vi "MCSC_4CH_4.04.vi"() -> ()   [LabVIEW 2012]
uses:
  <vilib>/Analysis/baseanly.llb/Mean (DBL).vi
  Libraries and VIs/Scalar_Data_4.vi
  Libraries and VIs/Scalar_Data_3.vi
  Libraries and VIs/Scalar_Data_2.vi
  Libraries and VIs/Scalar_Data.vi
  AmcsUsb.dll
  <vilib>/Analysis/NI_AALBase.lvlib
panel:
  in  "y":dbl
  in  "Data Reads":i32=962
  out "Loop Count":i32=961
  in  "TC Start":i32=100 min=100 max=1894
  in  "TC Length":i32=1894 min=100 max=1894
  out "Total Counts":cluster{dbl, dbl, dbl, dbl}(graph)={27003.0, 22784.0, 0.0, 0.0}
  out "return type":i32
  out "Raw Uncorrected Return":dbl[][](graph)=[[20897.0, 50029.0, 450.0, 783.0, 1128.0, 1525.0, 1812.0, 1978.0, 1912.0, 1724.0, 1571.0, 1324.0, 1184.0, 1034.0, 915.0, 833.0, 773.0, 692.0, 623.0, 619.0, 486.0, 513.0, 479.0, 406.0, 417.0, 375.0, 341.0, 359.0, 321.0, 307.0, 290.0, 262.0, 248.0, 258.0, 190.0, 213.0, 203.0, 200.0, 203.0, 201.0, 156.0, 159.0, 181.0, 160.0, 179.0, 176.0, 175.0, 192.0, 163.0, 145.0, 185.0, 176.0, 166.0, 155.0, 167.0, 159.0, 149.0, 154.0, 232.0, 335.0, 318.0, 198.0, 164.0, 167.0, 148.0, 145.0, 151.0, 129.0, 173.0, 165.0, 139.0, 150.0, 165.0, 157.0, 165.0, 158.0, 144.0, 160.0, 163.0, 159.0, 146.0, 139.0, 136.0, 134.0, 168.0, 141.0, 123.0, 160.0, 142.0, 151.0, 159.0, 167.0, 145.0, 160.0, 154.0, 144.0, 150.0, 157.0, 146.0, 146.0, 143.0, 171.0, 165.0, 142.0, 149.0, 150.0, 158.0, 148.0, 153.0, 142.0, 142.0, 141.0, 174.0, 141.0, 161.0, 163.0, 144.0, 134.0, 136.0, 142.0, 148.0, 140.0, 157.0, 172.0, 167.0, 152.0, 147.0, 137.0, 166.0, 149.0, 135.0, 132.0, 142.0, 142.0, 140.0, 148.0, 163.0, 160.0, 130.0, 130.0, 162.0, 174.0, 153.0, 157.0, 154.0, 171.0, 152.0, 160.0, 150.0, 180.0, 139.0, 140.0, 156.0, 148.0, 141.0, 158.0, 157.0, 133.0, 166.0, 146.0, 146.0, 150.0, 138.0, 133.0, 165.0, 153.0, 133.0, 128.0, 129.0, 157.0, 154.0, 136.0, 145.0, 159.0, 142.0, 131.0, 133.0, 148.0, 165.0, 143.0, 143.0, 135.0, 134.0, 151.0, 179.0, 166.0, 144.0, 151.0, 166.0, 152.0, 156.0, 150.0, 160.0, 130.0, 164.0, 147.0, 155.0, 129.0, 164.0, 163.0, 163.0, 133.0, 182.0, 153.0, 128.0, 151.0, 157.0, 144.0, 180.0, 129.0, 148.0, 136.0, 144.0, 150.0, 146.0, 145.0, 163.0, 146.0, 158.0, 150.0, 154.0, 180.0, 152.0, 152.0, 153.0, 148.0, 158.0, 152.0, 161.0, 154.0, 151.0, 124.0, 133.0, 143.0, 154.0, 134.0, 144.0, 152.0, 150.0, 161.0, 148.0, 156.0, 129.0, 162.0, 157.0, 154.0, 167.0, 149.0, 159.0, 170.0, 155.0, 158.0, 137.0, 149.0, 155.0, 149.0, 129.0, 156.0, 140.0, 170.0, 172.0, 149.0, 142.0, 153.0, 146.0, 152.0, 155.0, 143.0, 115.0, 135.0, 155.0, 145.0, 136.0, 154.0, 146.0, 161.0, 144.0, 170.0, 148.0, 137.0], [142.0, 41325.0, 486.0, 804.0, 1162.0, 1626.0, 1885.0, 1884.0, 1837.0, 1564.0, 1349.0, 1108.0, 1006.0, 860.0, 746.0, 643.0, 549.0, 466.0, 456.0, 433.0, 335.0, 343.0, 328.0, 255.0, 264.0, 235.0, 239.0, 222.0, 207.0, 180.0, 170.0, 159.0, 175.0, 169.0, 158.0, 168.0, 161.0, 154.0, 160.0, 166.0, 139.0, 124.0, 134.0, 165.0, 114.0, 120.0, 158.0, 144.0, 141.0, 127.0, 121.0, 126.0, 130.0, 128.0, 136.0, 115.0, 148.0, 132.0, 153.0, 178.0, 163.0, 145.0, 129.0, 124.0, 111.0, 115.0, 142.0, 128.0, 127.0, 157.0, 139.0, 135.0, 137.0, 148.0, 112.0, 119.0, 122.0, 137.0, 110.0, 140.0, 132.0, 135.0, 158.0, 151.0, 122.0, 123.0, 122.0, 130.0, 127.0, 134.0, 139.0, 140.0, 124.0, 116.0, 134.0, 129.0, 120.0, 138.0, 124.0, 129.0, 152.0, 115.0, 121.0, 113.0, 108.0, 126.0, 119.0, 133.0, 132.0, 134.0, 147.0, 126.0, 134.0, 101.0, 122.0, 130.0, 130.0, 128.0, 128.0, 131.0, 122.0, 118.0, 113.0, 135.0, 118.0, 128.0, 114.0, 128.0, 137.0, 148.0, 114.0, 116.0, 139.0, 129.0, 116.0, 123.0, 132.0, 128.0, 119.0, 123.0, 120.0, 115.0, 135.0, 127.0, 98.0, 115.0, 118.0, 110.0, 120.0, 100.0, 132.0, 131.0, 134.0, 126.0, 131.0, 131.0, 135.0, 116.0, 137.0, 131.0, 135.0, 118.0, 121.0, 109.0, 129.0, 126.0, 110.0, 85.0, 116.0, 126.0, 134.0, 122.0, 143.0, 132.0, 116.0, 136.0, 120.0, 128.0, 120.0, 130.0, 123.0, 139.0, 120.0, 112.0, 125.0, 123.0, 145.0, 127.0, 121.0, 141.0, 122.0, 128.0, 122.0, 127.0, 123.0, 119.0, 126.0, 133.0, 113.0, 124.0, 147.0, 126.0, 139.0, 124.0, 122.0, 108.0, 136.0, 129.0, 137.0, 151.0, 127.0, 129.0, 138.0, 104.0, 123.0, 132.0, 120.0, 132.0, 127.0, 132.0, 128.0, 123.0, 134.0, 137.0, 121.0, 135.0, 131.0, 123.0, 153.0, 134.0, 119.0, 120.0, 123.0, 124.0, 117.0, 116.0, 132.0, 120.0, 124.0, 135.0, 135.0, 131.0, 128.0, 132.0, 113.0, 133.0, 127.0, 136.0, 137.0, 116.0, 133.0, 132.0, 130.0, 131.0, 141.0, 127.0, 145.0, 127.0, 129.0, 112.0, 137.0, 126.0, 128.0, 134.0, 122.0, 137.0, 120.0, 131.0, 146.0, 153.0, 134.0, 125.0, 109.0, 110.0, 130.0, 134.0, 130.0, 128.0, 136.0, 126.0], [145.0, 0.0, 0.0, 0.0, 0.0, 0.0, 0.0, 0.0, 0.0, 0.0, 0.0, 0.0, 0.0, 0.0, 0.0, 0.0, 0.0, 0.0, 0.0, 0.0, 0.0, 0.0, 0.0, 0.0, 0.0, 0.0, 0.0, 0.0, 0.0, 0.0, 0.0, 0.0, 0.0, 0.0, 0.0, 0.0, 0.0, 0.0, 0.0, 0.0, 0.0, 0.0, 0.0, 0.0, 0.0, 0.0, 0.0, 0.0, 0.0, 0.0, 0.0, 0.0, 0.0, 0.0, 0.0, 0.0, 0.0, 0.0, 0.0, 0.0, 0.0, 0.0, 0.0, 0.0, 0.0, 0.0, 0.0, 0.0, 0.0, 0.0, 0.0, 0.0, 0.0, 0.0, 0.0, 0.0, 0.0, 0.0, 0.0, 0.0, 0.0, 0.0, 0.0, 0.0, 0.0, 0.0, 0.0, 0.0, 0.0, 0.0, 0.0, 0.0, 0.0, 0.0, 0.0, 0.0, 0.0, 0.0, 0.0, 0.0, 0.0, 0.0, 0.0, 0.0, 0.0, 0.0, 0.0, 0.0, 0.0, 0.0, 0.0, 0.0, 0.0, 0.0, 0.0, 0.0, 0.0, 0.0, 0.0, 0.0, 0.0, 0.0, 0.0, 0.0, 0.0, 0.0, 0.0, 0.0, 0.0, 0.0, 0.0, 0.0, 0.0, 0.0, 0.0, 0.0, 0.0, 0.0, 0.0, 0.0, 0.0, 0.0, 0.0, 0.0, 0.0, 0.0, 0.0, 0.0, 0.0, 0.0, 0.0, 0.0, 0.0, 0.0, 0.0, 0.0, 0.0, 0.0, 0.0, 0.0, 0.0, 0.0, 0.0, 0.0, 0.0, 0.0, 0.0, 0.0, 0.0, 0.0, 0.0, 0.0, 0.0, 0.0, 0.0, 0.0, 0.0, 0.0, 0.0, 0.0, 0.0, 0.0, 0.0, 0.0, 0.0, 0.0, 0.0, 0.0, 0.0, 0.0, 0.0, 0.0, 0.0, 0.0, 0.0, 0.0, 0.0, 0.0, 0.0, 0.0, 0.0, 0.0, 0.0, 0.0, 0.0, 0.0, 0.0, 0.0, 0.0, 0.0, 0.0, 0.0, 0.0, 0.0, 0.0, 0.0, 0.0, 0.0, 0.0, 0.0, 0.0, 0.0, 0.0, 0.0, 0.0, 0.0, 0.0, 0.0, 0.0, 0.0, 0.0, 0.0, 0.0, 0.0, 0.0, 0.0, 0.0, 0.0, 0.0, 0.0, 0.0, 0.0, 0.0, 0.0, 0.0, 0.0, 0.0, 0.0, 0.0, 0.0, 0.0, 0.0, 0.0, 0.0, 0.0, 0.0, 0.0, 0.0, 0.0, 0.0, 0.0, 0.0, 0.0, 0.0, 0.0, 0.0, 0.0, 0.0, 0.0, 0.0, 0.0, 0.0, 0.0, 0.0, 0.0, 0.0, 0.0, 0.0, 0.0, 0.0], [0.0, 0.0, 0.0, 0.0, 0.0, 0.0, 0.0, 0.0, 0.0, 0.0, 0.0, 0.0, 0.0, 0.0, 0.0, 0.0, 0.0, 0.0, 0.0, 0.0, 0.0, 0.0, 0.0, 0.0, 0.0, 0.0, 0.0, 0.0, 0.0, 0.0, 0.0, 0.0, 0.0, 0.0, 0.0, 0.0, 0.0, 0.0, 0.0, 0.0, 0.0, 0.0, 0.0, 0.0, 0.0, 0.0, 0.0, 0.0, 0.0, 0.0, 0.0, 0.0, 0.0, 0.0, 0.0, 0.0, 0.0, 0.0, 0.0, 0.0, 0.0, 0.0, 0.0, 0.0, 0.0, 0.0, 0.0, 0.0, 0.0, 0.0, 0.0, 0.0, 0.0, 0.0, 0.0, 0.0, 0.0, 0.0, 0.0, 0.0, 0.0, 0.0, 0.0, 0.0, 0.0, 0.0, 0.0, 0.0, 0.0, 0.0, 0.0, 0.0, 0.0, 0.0, 0.0, 0.0, 0.0, 0.0, 0.0, 0.0, 0.0, 0.0, 0.0, 0.0, 0.0, 0.0, 0.0, 0.0, 0.0, 0.0, 0.0, 0.0, 0.0, 0.0, 0.0, 0.0, 0.0, 0.0, 0.0, 0.0, 0.0, 0.0, 0.0, 0.0, 0.0, 0.0, 0.0, 0.0, 0.0, 0.0, 0.0, 0.0, 0.0, 0.0, 0.0, 0.0, 0.0, 0.0, 0.0, 0.0, 0.0, 0.0, 0.0, 0.0, 0.0, 0.0, 0.0, 0.0, 0.0, 0.0, 0.0, 0.0, 0.0, 0.0, 0.0, 0.0, 0.0, 0.0, 0.0, 0.0, 0.0, 0.0, 0.0, 0.0, 0.0, 0.0, 0.0, 0.0, 0.0, 0.0, 0.0, 0.0, 0.0, 0.0, 0.0, 0.0, 0.0, 0.0, 0.0, 0.0, 0.0, 0.0, 0.0, 0.0, 0.0, 0.0, 0.0, 0.0, 0.0, 0.0, 0.0, 0.0, 0.0, 0.0, 0.0, 0.0, 0.0, 0.0, 0.0, 0.0, 0.0, 0.0, 0.0, 0.0, 0.0, 0.0, 0.0, 0.0, 0.0, 0.0, 0.0, 0.0, 0.0, 0.0, 0.0, 0.0, 0.0, 0.0, 0.0, 0.0, 0.0, 0.0, 0.0, 0.0, 0.0, 0.0, 0.0, 0.0, 0.0, 0.0, 0.0, 0.0, 0.0, 0.0, 0.0, 0.0, 0.0, 0.0, 0.0, 0.0, 0.0, 0.0, 0.0, 0.0, 0.0, 0.0, 0.0, 0.0, 0.0, 0.0, 0.0, 0.0, 0.0, 0.0, 0.0, 0.0, 0.0, 0.0, 0.0, 0.0, 0.0, 0.0, 0.0, 0.0, 0.0, 0.0, 0.0, 0.0, 0.0, 0.0, 0.0, 0.0, 0.0, 0.0, 0.0, 0.0, 0.0, 0.0, 0.0, 0.0]]
  in  "stop":bool
  out "Corrected Return":dbl[][](graph)=[[20749.1, 49881.1, 302.1, 635.1, 980.1, 1377.1, 1664.1, 1830.1, 1764.1, 1576.1, 1423.1, 1176.1, 1036.1, 886.1, 767.1, 685.1, 625.1, 544.1, 475.1, 471.1, 338.1, 365.1, 331.1, 258.1, 269.1, 227.1, 193.1, 211.1, 173.1, 159.1, 142.1, 114.1, 100.1, 110.1, 42.099999999999994, 65.1, 55.099999999999994, 52.099999999999994, 55.099999999999994, 53.099999999999994, 8.099999999999994, 11.099999999999994, 33.099999999999994, 12.099999999999994, 31.099999999999994, 28.099999999999994, 27.099999999999994, 44.099999999999994, 15.099999999999994, -2.9000000000000057, 37.099999999999994, 28.099999999999994, 18.099999999999994, 7.099999999999994, 19.099999999999994, 11.099999999999994, 1.0999999999999943, 6.099999999999994, 84.1, 187.1, 170.1, 50.099999999999994, 16.099999999999994, 19.099999999999994, 0.09999999999999432, -2.9000000000000057, 3.0999999999999943, -18.900000000000006, 25.099999999999994, 17.099999999999994, -8.900000000000006, 2.0999999999999943, 17.099999999999994, 9.099999999999994, 17.099999999999994, 10.099999999999994, -3.9000000000000057, 12.099999999999994, 15.099999999999994, 11.099999999999994, -1.9000000000000057, -8.900000000000006, -11.900000000000006, -13.900000000000006, 20.099999999999994, -6.900000000000006, -24.900000000000006, 12.099999999999994, -5.900000000000006, 3.0999999999999943, 11.099999999999994, 19.099999999999994, -2.9000000000000057, 12.099999999999994, 6.099999999999994, -3.9000000000000057, 2.0999999999999943, 9.099999999999994, -1.9000000000000057, -1.9000000000000057, -4.900000000000006, 23.099999999999994, 17.099999999999994, -5.900000000000006, 1.0999999999999943, 2.0999999999999943, 10.099999999999994, 0.09999999999999432, 5.099999999999994, -5.900000000000006, -5.900000000000006, -6.900000000000006, 26.099999999999994, -6.900000000000006, 13.099999999999994, 15.099999999999994, -3.9000000000000057, -13.900000000000006, -11.900000000000006, -5.900000000000006, 0.09999999999999432, -7.900000000000006, 9.099999999999994, 24.099999999999994, 19.099999999999994, 4.099999999999994, -0.9000000000000057, -10.900000000000006, 18.099999999999994, 1.0999999999999943, -12.900000000000006, -15.900000000000006, -5.900000000000006, -5.900000000000006, -7.900000000000006, 0.09999999999999432, 15.099999999999994, 12.099999999999994, -17.900000000000006, -17.900000000000006, 14.099999999999994, 26.099999999999994, 5.099999999999994, 9.099999999999994, 6.099999999999994, 23.099999999999994, 4.099999999999994, 12.099999999999994, 2.0999999999999943, 32.099999999999994, -8.900000000000006, -7.900000000000006, 8.099999999999994, 0.09999999999999432, -6.900000000000006, 10.099999999999994, 9.099999999999994, -14.900000000000006, 18.099999999999994, -1.9000000000000057, -1.9000000000000057, 2.0999999999999943, -9.900000000000006, -14.900000000000006, 17.099999999999994, 5.099999999999994, -14.900000000000006, -19.900000000000006, -18.900000000000006, 9.099999999999994, 6.099999999999994, -11.900000000000006, -2.9000000000000057, 11.099999999999994, -5.900000000000006, -16.900000000000006, -14.900000000000006, 0.09999999999999432, 17.099999999999994, -4.900000000000006, -4.900000000000006, -12.900000000000006, -13.900000000000006, 3.0999999999999943, 31.099999999999994, 18.099999999999994, -3.9000000000000057, 3.0999999999999943, 18.099999999999994, 4.099999999999994, 8.099999999999994, 2.0999999999999943, 12.099999999999994, -17.900000000000006, 16.099999999999994, -0.9000000000000057, 7.099999999999994, -18.900000000000006, 16.099999999999994, 15.099999999999994, 15.099999999999994, -14.900000000000006, 34.099999999999994, 5.099999999999994, -19.900000000000006, 3.0999999999999943, 9.099999999999994, -3.9000000000000057, 32.099999999999994, -18.900000000000006, 0.09999999999999432, -11.900000000000006, -3.9000000000000057, 2.0999999999999943, -1.9000000000000057, -2.9000000000000057, 15.099999999999994, -1.9000000000000057, 10.099999999999994, 2.0999999999999943, 6.099999999999994, 32.099999999999994, 4.099999999999994, 4.099999999999994, 5.099999999999994, 0.09999999999999432, 10.099999999999994, 4.099999999999994, 13.099999999999994, 6.099999999999994, 3.0999999999999943, -23.900000000000006, -14.900000000000006, -4.900000000000006, 6.099999999999994, -13.900000000000006, -3.9000000000000057, 4.099999999999994, 2.0999999999999943, 13.099999999999994, 0.09999999999999432, 8.099999999999994, -18.900000000000006, 14.099999999999994, 9.099999999999994, 6.099999999999994, 19.099999999999994, 1.0999999999999943, 11.099999999999994, 22.099999999999994, 7.099999999999994, 10.099999999999994, -10.900000000000006, 1.0999999999999943, 7.099999999999994, 1.0999999999999943, -18.900000000000006, 8.099999999999994, -7.900000000000006, 22.099999999999994, 24.099999999999994, 1.0999999999999943, -5.900000000000006, 5.099999999999994, -1.9000000000000057, 4.099999999999994, 7.099999999999994, -4.900000000000006, -32.900000000000006, -12.900000000000006, 7.099999999999994, -2.9000000000000057, -11.900000000000006, 6.099999999999994, -1.9000000000000057, 13.099999999999994, -3.9000000000000057, 22.099999999999994, 0.09999999999999432, -10.900000000000006], [12.199999999999989, 41195.2, 356.2, 674.2, 1032.2, 1496.2, 1755.2, 1754.2, 1707.2, 1434.2, 1219.2, 978.2, 876.2, 730.2, 616.2, 513.2, 419.2, 336.2, 326.2, 303.2, 205.2, 213.2, 198.2, 125.19999999999999, 134.2, 105.19999999999999, 109.19999999999999, 92.19999999999999, 77.19999999999999, 50.19999999999999, 40.19999999999999, 29.19999999999999, 45.19999999999999, 39.19999999999999, 28.19999999999999, 38.19999999999999, 31.19999999999999, 24.19999999999999, 30.19999999999999, 36.19999999999999, 9.199999999999989, -5.800000000000011, 4.199999999999989, 35.19999999999999, -15.800000000000011, -9.800000000000011, 28.19999999999999, 14.199999999999989, 11.199999999999989, -2.8000000000000114, -8.800000000000011, -3.8000000000000114, 0.19999999999998863, -1.8000000000000114, 6.199999999999989, -14.800000000000011, 18.19999999999999, 2.1999999999999886, 23.19999999999999, 48.19999999999999, 33.19999999999999, 15.199999999999989, -0.8000000000000114, -5.800000000000011, -18.80000000000001, -14.800000000000011, 12.199999999999989, -1.8000000000000114, -2.8000000000000114, 27.19999999999999, 9.199999999999989, 5.199999999999989, 7.199999999999989, 18.19999999999999, -17.80000000000001, -10.800000000000011, -7.800000000000011, 7.199999999999989, -19.80000000000001, 10.199999999999989, 2.1999999999999886, 5.199999999999989, 28.19999999999999, 21.19999999999999, -7.800000000000011, -6.800000000000011, -7.800000000000011, 0.19999999999998863, -2.8000000000000114, 4.199999999999989, 9.199999999999989, 10.199999999999989, -5.800000000000011, -13.800000000000011, 4.199999999999989, -0.8000000000000114, -9.800000000000011, 8.199999999999989, -5.800000000000011, -0.8000000000000114, 22.19999999999999, -14.800000000000011, -8.800000000000011, -16.80000000000001, -21.80000000000001, -3.8000000000000114, -10.800000000000011, 3.1999999999999886, 2.1999999999999886, 4.199999999999989, 17.19999999999999, -3.8000000000000114, 4.199999999999989, -28.80000000000001, -7.800000000000011, 0.19999999999998863, 0.19999999999998863, -1.8000000000000114, -1.8000000000000114, 1.1999999999999886, -7.800000000000011, -11.800000000000011, -16.80000000000001, 5.199999999999989, -11.800000000000011, -1.8000000000000114, -15.800000000000011, -1.8000000000000114, 7.199999999999989, 18.19999999999999, -15.800000000000011, -13.800000000000011, 9.199999999999989, -0.8000000000000114, -13.800000000000011, -6.800000000000011, 2.1999999999999886, -1.8000000000000114, -10.800000000000011, -6.800000000000011, -9.800000000000011, -14.800000000000011, 5.199999999999989, -2.8000000000000114, -31.80000000000001, -14.800000000000011, -11.800000000000011, -19.80000000000001, -9.800000000000011, -29.80000000000001, 2.1999999999999886, 1.1999999999999886, 4.199999999999989, -3.8000000000000114, 1.1999999999999886, 1.1999999999999886, 5.199999999999989, -13.800000000000011, 7.199999999999989, 1.1999999999999886, 5.199999999999989, -11.800000000000011, -8.800000000000011, -20.80000000000001, -0.8000000000000114, -3.8000000000000114, -19.80000000000001, -44.80000000000001, -13.800000000000011, -3.8000000000000114, 4.199999999999989, -7.800000000000011, 13.199999999999989, 2.1999999999999886, -13.800000000000011, 6.199999999999989, -9.800000000000011, -1.8000000000000114, -9.800000000000011, 0.19999999999998863, -6.800000000000011, 9.199999999999989, -9.800000000000011, -17.80000000000001, -4.800000000000011, -6.800000000000011, 15.199999999999989, -2.8000000000000114, -8.800000000000011, 11.199999999999989, -7.800000000000011, -1.8000000000000114, -7.800000000000011, -2.8000000000000114, -6.800000000000011, -10.800000000000011, -3.8000000000000114, 3.1999999999999886, -16.80000000000001, -5.800000000000011, 17.19999999999999, -3.8000000000000114, 9.199999999999989, -5.800000000000011, -7.800000000000011, -21.80000000000001, 6.199999999999989, -0.8000000000000114, 7.199999999999989, 21.19999999999999, -2.8000000000000114, -0.8000000000000114, 8.199999999999989, -25.80000000000001, -6.800000000000011, 2.1999999999999886, -9.800000000000011, 2.1999999999999886, -2.8000000000000114, 2.1999999999999886, -1.8000000000000114, -6.800000000000011, 4.199999999999989, 7.199999999999989, -8.800000000000011, 5.199999999999989, 1.1999999999999886, -6.800000000000011, 23.19999999999999, 4.199999999999989, -10.800000000000011, -9.800000000000011, -6.800000000000011, -5.800000000000011, -12.800000000000011, -13.800000000000011, 2.1999999999999886, -9.800000000000011, -5.800000000000011, 5.199999999999989, 5.199999999999989, 1.1999999999999886, -1.8000000000000114, 2.1999999999999886, -16.80000000000001, 3.1999999999999886, -2.8000000000000114, 6.199999999999989, 7.199999999999989, -13.800000000000011, 3.1999999999999886, 2.1999999999999886, 0.19999999999998863, 1.1999999999999886, 11.199999999999989, -2.8000000000000114, 15.199999999999989, -2.8000000000000114, -0.8000000000000114, -17.80000000000001, 7.199999999999989, -3.8000000000000114, -1.8000000000000114, 4.199999999999989, -7.800000000000011, 7.199999999999989, -9.800000000000011, 1.1999999999999886, 16.19999999999999, 23.19999999999999, 4.199999999999989, -4.800000000000011, -20.80000000000001, -19.80000000000001, 0.19999999999998863, 4.199999999999989, 0.19999999999998863, -1.8000000000000114, 6.199999999999989, -3.8000000000000114], [0.0, 0.0, 0.0, 0.0, 0.0, 0.0, 0.0, 0.0, 0.0, 0.0, 0.0, 0.0, 0.0, 0.0, 0.0, 0.0, 0.0, 0.0, 0.0, 0.0, 0.0, 0.0, 0.0, 0.0, 0.0, 0.0, 0.0, 0.0, 0.0, 0.0, 0.0, 0.0, 0.0, 0.0, 0.0, 0.0, 0.0, 0.0, 0.0, 0.0, 0.0, 0.0, 0.0, 0.0, 0.0, 0.0, 0.0, 0.0, 0.0, 0.0, 0.0, 0.0, 0.0, 0.0, 0.0, 0.0, 0.0, 0.0, 0.0, 0.0, 0.0, 0.0, 0.0, 0.0, 0.0, 0.0, 0.0, 0.0, 0.0, 0.0, 0.0, 0.0, 0.0, 0.0, 0.0, 0.0, 0.0, 0.0, 0.0, 0.0, 0.0, 0.0, 0.0, 0.0, 0.0, 0.0, 0.0, 0.0, 0.0, 0.0, 0.0, 0.0, 0.0, 0.0, 0.0, 0.0, 0.0, 0.0, 0.0, 0.0, 0.0, 0.0, 0.0, 0.0, 0.0, 0.0, 0.0, 0.0, 0.0, 0.0, 0.0, 0.0, 0.0, 0.0, 0.0, 0.0, 0.0, 0.0, 0.0, 0.0, 0.0, 0.0, 0.0, 0.0, 0.0, 0.0, 0.0, 0.0, 0.0, 0.0, 0.0, 0.0, 0.0, 0.0, 0.0, 0.0, 0.0, 0.0, 0.0, 0.0, 0.0, 0.0, 0.0, 0.0, 0.0, 0.0, 0.0, 0.0, 0.0, 0.0, 0.0, 0.0, 0.0, 0.0, 0.0, 0.0, 0.0, 0.0, 0.0, 0.0, 0.0, 0.0, 0.0, 0.0, 0.0, 0.0, 0.0, 0.0, 0.0, 0.0, 0.0, 0.0, 0.0, 0.0, 0.0, 0.0, 0.0, 0.0, 0.0, 0.0, 0.0, 0.0, 0.0, 0.0, 0.0, 0.0, 0.0, 0.0, 0.0, 0.0, 0.0, 0.0, 0.0, 0.0, 0.0, 0.0, 0.0, 0.0, 0.0, 0.0, 0.0, 0.0, 0.0, 0.0, 0.0, 0.0, 0.0, 0.0, 0.0, 0.0, 0.0, 0.0, 0.0, 0.0, 0.0, 0.0, 0.0, 0.0, 0.0, 0.0, 0.0, 0.0, 0.0, 0.0, 0.0, 0.0, 0.0, 0.0, 0.0, 0.0, 0.0, 0.0, 0.0, 0.0, 0.0, 0.0, 0.0, 0.0, 0.0, 0.0, 0.0, 0.0, 0.0, 0.0, 0.0, 0.0, 0.0, 0.0, 0.0, 0.0, 0.0, 0.0, 0.0, 0.0, 0.0, 0.0, 0.0, 0.0, 0.0, 0.0, 0.0, 0.0, 0.0, 0.0, 0.0, 0.0, 0.0, 0.0, 0.0, 0.0, 0.0, 0.0, 0.0, 0.0, 0.0, 0.0, 0.0, 0.0, 0.0, 0.0], [0.0, 0.0, 0.0, 0.0, 0.0, 0.0, 0.0, 0.0, 0.0, 0.0, 0.0, 0.0, 0.0, 0.0, 0.0, 0.0, 0.0, 0.0, 0.0, 0.0, 0.0, 0.0, 0.0, 0.0, 0.0, 0.0, 0.0, 0.0, 0.0, 0.0, 0.0, 0.0, 0.0, 0.0, 0.0, 0.0, 0.0, 0.0, 0.0, 0.0, 0.0, 0.0, 0.0, 0.0, 0.0, 0.0, 0.0, 0.0, 0.0, 0.0, 0.0, 0.0, 0.0, 0.0, 0.0, 0.0, 0.0, 0.0, 0.0, 0.0, 0.0, 0.0, 0.0, 0.0, 0.0, 0.0, 0.0, 0.0, 0.0, 0.0, 0.0, 0.0, 0.0, 0.0, 0.0, 0.0, 0.0, 0.0, 0.0, 0.0, 0.0, 0.0, 0.0, 0.0, 0.0, 0.0, 0.0, 0.0, 0.0, 0.0, 0.0, 0.0, 0.0, 0.0, 0.0, 0.0, 0.0, 0.0, 0.0, 0.0, 0.0, 0.0, 0.0, 0.0, 0.0, 0.0, 0.0, 0.0, 0.0, 0.0, 0.0, 0.0, 0.0, 0.0, 0.0, 0.0, 0.0, 0.0, 0.0, 0.0, 0.0, 0.0, 0.0, 0.0, 0.0, 0.0, 0.0, 0.0, 0.0, 0.0, 0.0, 0.0, 0.0, 0.0, 0.0, 0.0, 0.0, 0.0, 0.0, 0.0, 0.0, 0.0, 0.0, 0.0, 0.0, 0.0, 0.0, 0.0, 0.0, 0.0, 0.0, 0.0, 0.0, 0.0, 0.0, 0.0, 0.0, 0.0, 0.0, 0.0, 0.0, 0.0, 0.0, 0.0, 0.0, 0.0, 0.0, 0.0, 0.0, 0.0, 0.0, 0.0, 0.0, 0.0, 0.0, 0.0, 0.0, 0.0, 0.0, 0.0, 0.0, 0.0, 0.0, 0.0, 0.0, 0.0, 0.0, 0.0, 0.0, 0.0, 0.0, 0.0, 0.0, 0.0, 0.0, 0.0, 0.0, 0.0, 0.0, 0.0, 0.0, 0.0, 0.0, 0.0, 0.0, 0.0, 0.0, 0.0, 0.0, 0.0, 0.0, 0.0, 0.0, 0.0, 0.0, 0.0, 0.0, 0.0, 0.0, 0.0, 0.0, 0.0, 0.0, 0.0, 0.0, 0.0, 0.0, 0.0, 0.0, 0.0, 0.0, 0.0, 0.0, 0.0, 0.0, 0.0, 0.0, 0.0, 0.0, 0.0, 0.0, 0.0, 0.0, 0.0, 0.0, 0.0, 0.0, 0.0, 0.0, 0.0, 0.0, 0.0, 0.0, 0.0, 0.0, 0.0, 0.0, 0.0, 0.0, 0.0, 0.0, 0.0, 0.0, 0.0, 0.0, 0.0, 0.0, 0.0, 0.0, 0.0, 0.0, 0.0, 0.0, 0.0, 0.0, 0.0, 0.0, 0.0, 0.0, 0.0]] caption="Corrected Signal"
  out "Max. Rep. Rate (Hz)":dbl=7091.695624423801
  out "Data Collection Time per Column":dbl=1.4001
  out "Minimum Sync Pulse Period(µs)":dbl=141.01 format="%.2f"
  in  "y units":u16(ring) items=["Bin #", "Sampling Time(µs)", "Range(m)"]
  in  "Time Resolution Per Bin(ns)":u16=500 min=5 max=1063 step=1
  in  "Number of Accumulates":u32=10000 min=1 max=32767 step=1
  in  "Number of Bins":u32=280 min=2 max=4095 step=1
  in  "Pulse A Polarity":enum16{"Low", "High"}(ring)=enum."High"
  in  "Sync Pulse Polarity":enum32{"Low", "High"}(ring)=enum."High"
  in  "Accumulation Delay(ns)":u16=10 min=10 max=1270 step=1
  in  "Pulse B Delay(ns)":u32=170000 min=80 max=327600 step=1
  in  "Pulse A Delay(ns)":u32=1040 min=80 max=327600
  in  "bins":u32=280 min=2 max=4095 step=1
  out "y offset":u16=10
  in  "ns scale":u16=500
  in  "Pulse B Polarity":enum16{"Low", "High"}(ring)=enum."High"
  out "Running?":bool
  out "Device ID":u32
  out "Open?":bool=TRUE
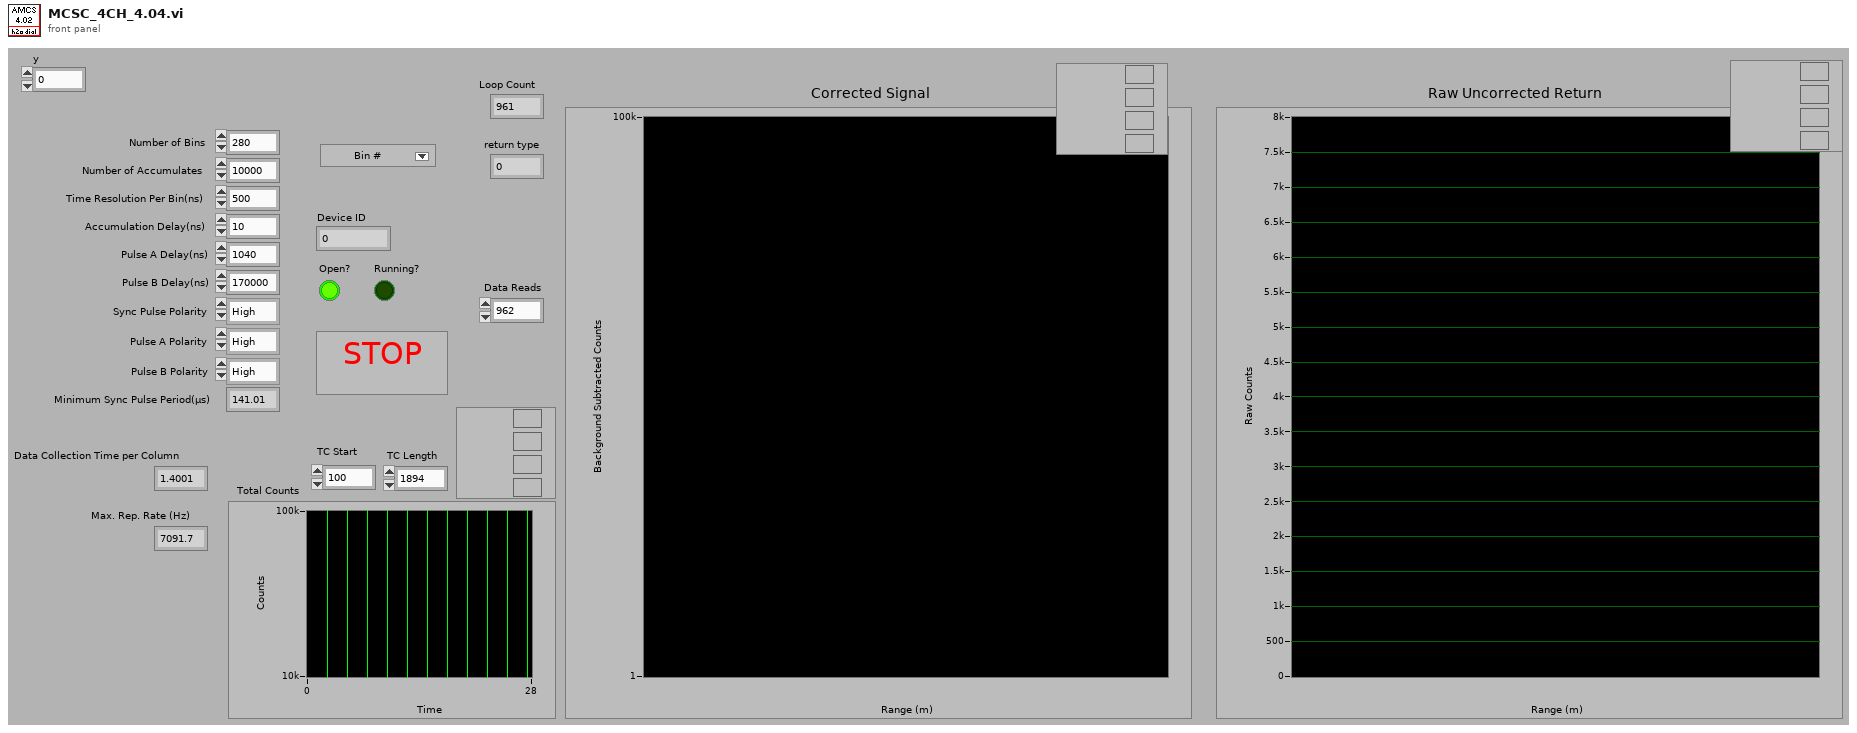
[diagram p1: front panel]
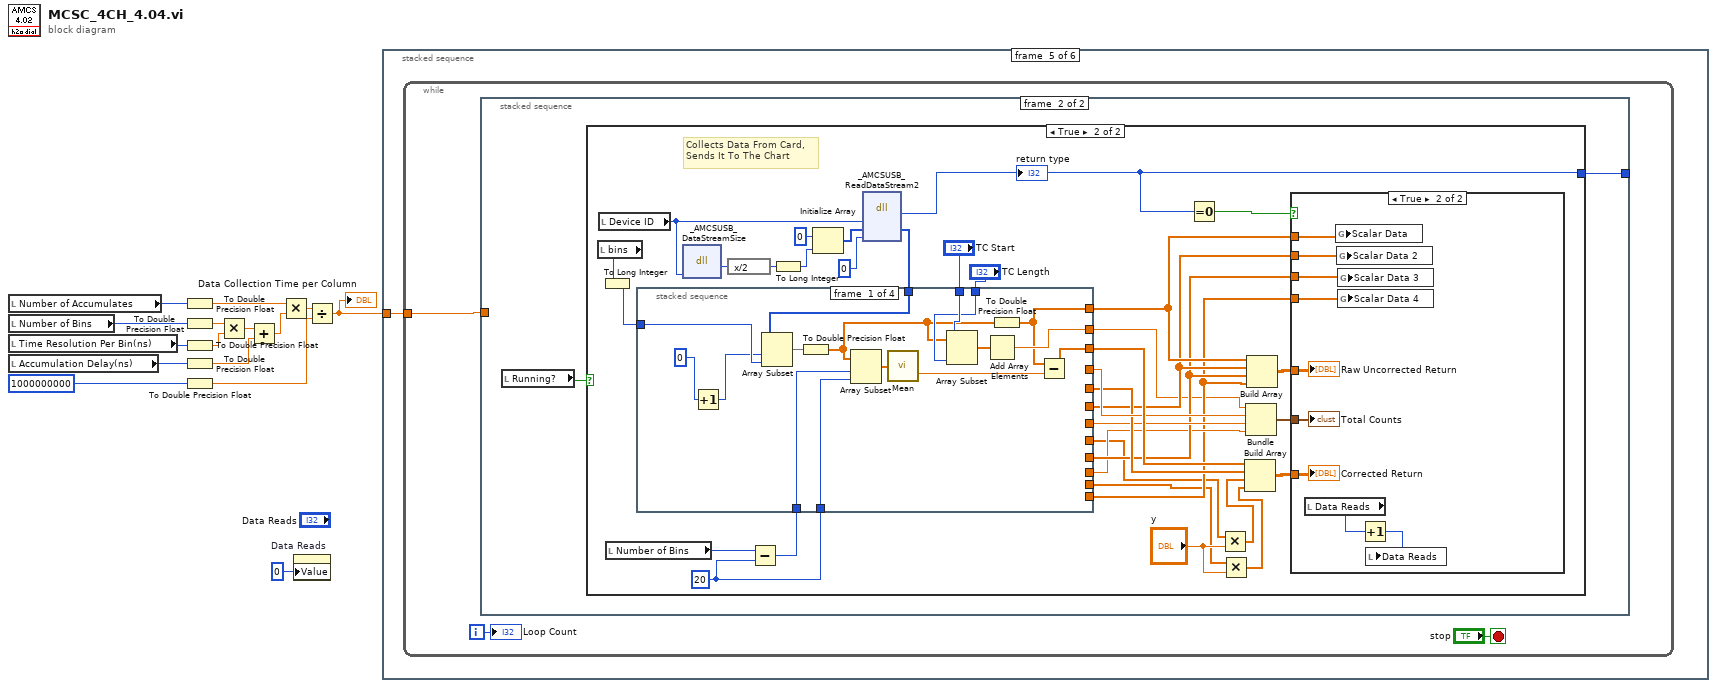
[diagram p0: block diagram]
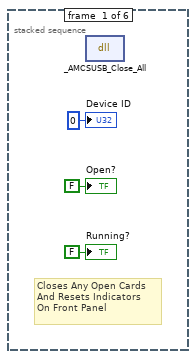
[diagram p2: hidden frame]
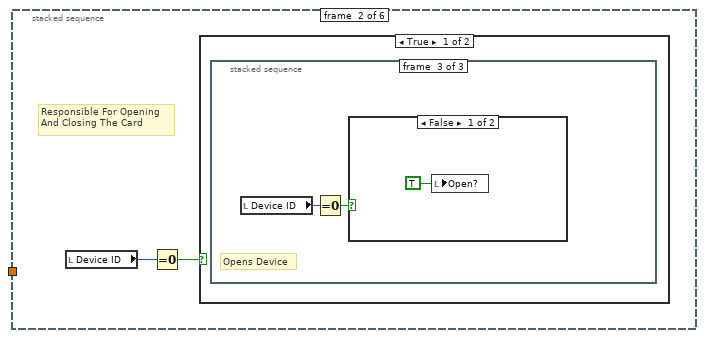
[diagram p3: hidden frame]
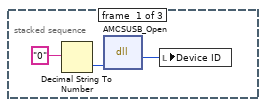
[diagram p4: hidden frame]
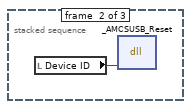
[diagram p5: hidden frame]
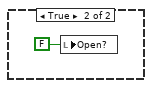
[diagram p6: hidden frame]
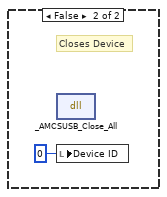
[diagram p7: hidden frame]
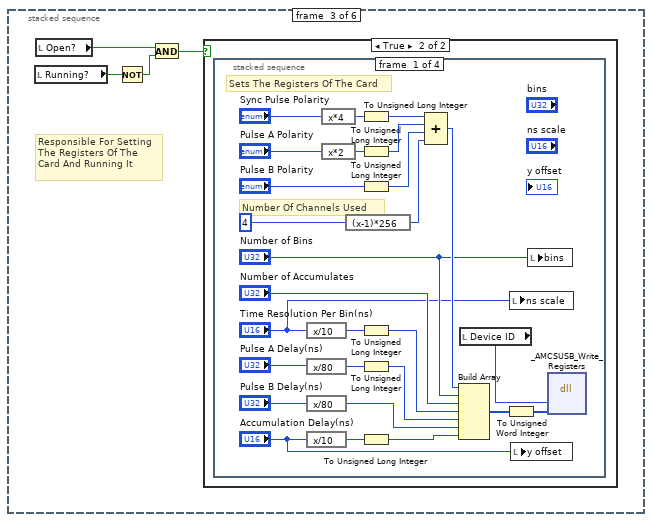
[diagram p8: hidden frame]
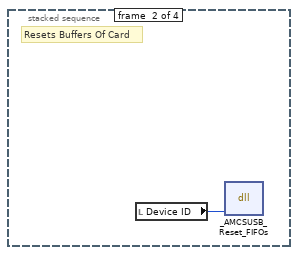
[diagram p10: hidden frame]
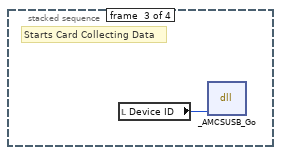
[diagram p11: hidden frame]
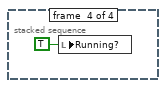
[diagram p12: hidden frame]
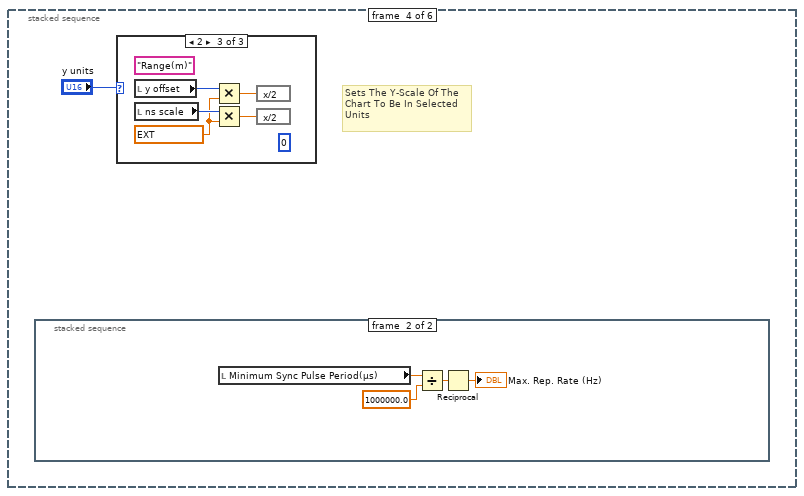
[diagram p13: hidden frame]
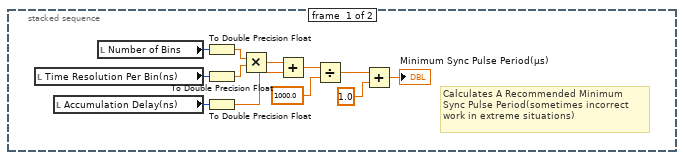
[diagram p14: hidden frame]
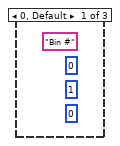
[diagram p15: hidden frame]
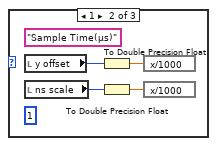
[diagram p16: hidden frame]
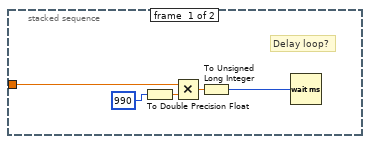
[diagram p17: hidden frame]
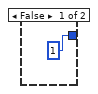
[diagram p18: hidden frame]
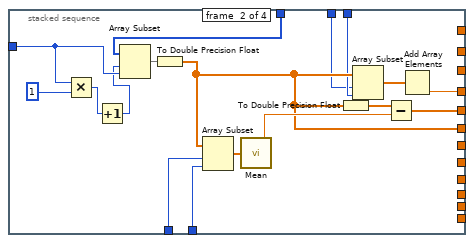
[diagram p20: hidden frame]
diagram:
  n1 = local read "Number of Accumulates"() -> (w11:u32)
  n2 = local read "Number of Bins"() -> (w6:u32)
  n3 = local read "Time Resolution Per Bin(ns)"() -> (w4:u16)
  n4 = local read "Accumulation Delay(ns)"() -> (w2:u16)
  n5 = To Double Precision Float(number=w11) -> (double precision float=w10:dbl)
  n6 = To Double Precision Float(number=w6) -> (double precision float=w5:dbl)
  n7 = To Double Precision Float(number=w4) -> (double precision float=w7:dbl)
  n8 = To Double Precision Float(number=w2) -> (double precision float=w3:dbl)
  n9 = To Double Precision Float(number=1000000000) -> (double precision float=w8:dbl)
  n10 = Multiply(x=w5, y=w7) -> (x*y=w15:dbl)
  n11 = Add(x=w15, y=w3) -> (x+y=w14:dbl)
  n12 = Multiply(x=w10, y=w14) -> (x*y=w13:dbl)
  n13 = property on="Data Reads" class="DigNum (strict)"("Value"=0 ("Data Reads")) -> ()  [unwired: 2 in, 2 out]
  n14 = Divide(x=w13, y=w8) -> (x/y=w12:dbl)
  "Data Collection Time per Column" <- w12
  n15 = stacked-sequence {
    tunnel: w12 -> [_ _ _ _ w90 _]
    frame #0 {
      # "Closes Any Open Cards\nAnd Resets Indicators\nOn Front Panel"
      n16 = dll-call lib="AmcsUsb.dll" fn="_AMCSUSB_Close_All" label="Close_All"() -> ()  [unwired: 4 in, 2 out]
      "Open?" <- FALSE ("Open?")
      "Device ID" <- u32 0 ("Device ID")
      "Running?" <- FALSE ("Running?")
    }
    frame #1 {
      # "Responsible For Opening\nAnd Closing The Card"
      n17 = local read "Device ID"() -> (w20:u32)
      n18 = Equal To 0?(x=w20) -> (x = 0?=w19:bool)
      n19 = case shown="True" w19 {
        frame True {
          # "Opens Device"
          n20 = stacked-sequence {
            frame #0 {
              n21 = Decimal String To Number(string="0" ("Device Number")) -> (number=w21:i32)  [unwired: 2 in, 1 out]
              n22 = dll-call lib="AmcsUsb.dll" fn="AMCSUSB_Open"("devnum"=w21) -> ("return type"=w22:u32)  [unwired: 4 in, 2 out]
              n23 = local write "Device ID"(w22) -> ()
            }
            frame #1 {
              n24 = local read "Device ID"() -> (w24:u32)
              n25 = dll-call lib="AmcsUsb.dll" fn="_AMCSUSB_Reset" label="Reset"("handle"=w24) -> ()  [unwired: 5 in, 2 out]
            }
            frame #2 {
              n26 = local read "Device ID"() -> (w25:u32)
              n27 = Equal To 0?(x=w25) -> (x = 0?=w26:bool)
              n28 = case shown="False" w26 {
                frame False {
                  n29 = local write "Open?"(TRUE ("Open?")) -> ()
                }
                frame True {
                  n30 = local write "Open?"(FALSE ("Open?")) -> ()
                }
              }
            }
          }
        }
        frame False {
          # "Closes Device"
          n31 = dll-call lib="AmcsUsb.dll" fn="_AMCSUSB_Close_All" label="Close_All"() -> ()  [unwired: 4 in, 2 out]
          n32 = local write "Device ID"(u32 0 ("Device ID")) -> ()
        }
      }
    }
    frame #2 {
      # "Responsible For Setting\nThe Registers Of The\nCard And Running It"
      n33 = local read "Running?"() -> (w32:bool)
      n34 = local read "Open?"() -> (w33:bool)
      n35 = Not(x=w32) -> (.not. x?=w31:bool)
      n36 = And(x=w33, y=w31) -> (x .and. y?=w30:bool)
      n37 = case shown="True" w30 {
        frame False {
        }
        frame True {
          n38 = stacked-sequence {
            frame #0 {
              # "Sets The Registers Of The Card"
              # "Number Of Channels Used"
              n39 = expression code="x/10"("Time Resolution Per Bin(ns)") -> (w37:u16)
              n40 = expression code="x/80"("Pulse A Delay(ns)") -> (w39:u32)
              n41 = expression code="x/80"("Pulse B Delay(ns)") -> (w60:u32)
              n42 = expression code="x/10"("Accumulation Delay(ns)") -> (w41:u16)
              n43 = expression code="x*4"("Sync Pulse Polarity") -> (w46:enum32{"Low", "High"})
              n44 = expression code="x*2"("Pulse A Polarity") -> (w45:enum16{"Low", "High"})
              n45 = expression code="(x-1)*256"(u32 4 ("Number of Channels Used")) -> (w54:u32)
              n46 = To Unsigned Long Integer(number=w46) -> (unsigned 32bit integer=w47:u32)
              n47 = To Unsigned Long Integer(number=w45) -> (unsigned 32bit integer=w44:u32)
              n48 = To Unsigned Long Integer(number="Pulse B Polarity") -> (unsigned 32bit integer=w42:u32)
              n49 = To Unsigned Long Integer(number=w37) -> (unsigned 32bit integer=w36:u32)
              n50 = To Unsigned Long Integer(number=w39) -> (unsigned 32bit integer=w38:u32)
              n51 = To Unsigned Long Integer(number=w41) -> (unsigned 32bit integer=w40:u32)
              n52 = Compound Arithmetic op=ADD(w47, w44, w42, w54) -> (w59:u32)
              n53 = Build Array(w59, "Number of Bins", "Number of Accumulates", w36, w38, w60, w40) -> (w35:u32[])
              n54 = local read "Device ID"() -> (w52:u32)
              n55 = To Unsigned Word Integer(number=w35) -> (unsigned 16bit integer=w34:u16[])
              n56 = local write "ns scale"("Time Resolution Per Bin(ns)") -> ()
              n57 = local write "y offset"("Accumulation Delay(ns)") -> ()
              n58 = local write "bins"("Number of Bins") -> ()
              n59 = dll-call lib="AmcsUsb.dll" fn="_AMCSUSB_Write_Registers" label="Write_Registers"("handle"=w52, "registers"=w34) -> ()  [unwired: 6 in, 2 out]
            }
            frame #1 {
              # "Resets Buffers Of Card"
              n60 = local read "Device ID"() -> (w61:u32)
              n61 = dll-call lib="AmcsUsb.dll" fn="_AMCSUSB_Reset_FIFOs" label="Reset_FIFOs"("handle"=w61) -> ()  [unwired: 5 in, 2 out]
            }
            frame #2 {
              # "Starts Card Collecting Data"
              n62 = local read "Device ID"() -> (w62:u32)
              n63 = dll-call lib="AmcsUsb.dll" fn="_AMCSUSB_Go" label="Go"("handle"=w62) -> ()  [unwired: 5 in, 2 out]
            }
            frame #3 {
              n64 = local write "Running?"(TRUE) -> ()
            }
          }
        }
      }
    }
    frame #3 {
      # "Sets The Y-Scale Of The\nChart To Be In Selected\nUnits"
      n65 = stacked-sequence {
        frame #0 {
          # "Calculates A Recommended Minimum\nSync Pulse Period(sometimes incorrect\nwork in extreme situations)"
          n66 = local read "Time Resolution Per Bin(ns)"() -> (w71:u16)
          n67 = local read "Accumulation Delay(ns)"() -> (w73:u16)
          n68 = local read "Number of Bins"() -> (w72:u32)
          n69 = To Double Precision Float(number=w72) -> (double precision float=w74:dbl)
          n70 = To Double Precision Float(number=w71) -> (double precision float=w75:dbl)
          n71 = To Double Precision Float(number=w73) -> (double precision float=w76:dbl)
          n72 = Multiply(x=w74, y=w75) -> (x*y=w70:dbl)
          n73 = Add(x=w70, y=w76) -> (x+y=w68:dbl)
          n74 = Divide(x=w68, y=1000.0) -> (x/y=w67:dbl)
          n75 = Add(x=w67, y=1.0) -> (x+y=→"Minimum Sync Pulse Period(µs)":dbl)
        }
        frame #1 {
          n76 = local read "Minimum Sync Pulse Period(µs)"() -> (w78:dbl)
          n77 = Divide(x=w78, y=1000000.0) -> (x/y=w77:dbl)
          n78 = Reciprocal(x=w77) -> (1/x=→"Max. Rep. Rate (Hz)":dbl)
        }
      }
      n79 = case shown="2" "y units" {
        frame 0, Default {
          (unwired) u8 0 ("Y Scale.Format & Precision:Precision")
          (unwired) u16 1 ("Y Scale.Offset and Multiplier:Multiplier")
          (unwired) "Bin #" ("Y Scale.Name Label.Text")
          (unwired) u16 0 ("Y Scale.Offset and Multiplier:Offset")
        }
        frame 1 {
          (unwired) u8 1 ("Y Scale.Format & Precision:Precision")
          (unwired) "Sample Time(µs)" ("Y Scale.Name Label.Text")
          n80 = local read "y offset"() -> (w84:u16)
          n81 = local read "ns scale"() -> (w83:u16)
          n82 = To Double Precision Float(number=w84) -> (double precision float=w82:dbl)
          n83 = To Double Precision Float(number=w83) -> (double precision float=w81:dbl)
          n84 = expression code="x/1000"(w82) -> ()  [unwired: 1 out]
          n85 = expression code="x/1000"(w81) -> ()  [unwired: 1 out]
        }
        frame 2 {
          (unwired) u8 0 ("Y Scale.Format & Precision:Precision")
          w85 = ext 0.299792458 ("y")
          (unwired) "Range(m)" ("Y Scale.Name Label.Text")
          n86 = local read "y offset"() -> (w88:u16)
          n87 = local read "ns scale"() -> (w89:u16)
          n88 = Multiply(x=w88, y=w85) -> (x*y=w87:ext)
          n89 = Multiply(x=w89, y=w85) -> (x*y=w86:ext)
          n90 = expression code="x/2"(w87) -> ()  [unwired: 1 out]
          n91 = expression code="x/2"(w86) -> ()  [unwired: 1 out]
        }
      }
    }
    frame #4 {
      n92 = while {
        tunnel: w90 -> [w93]
        i -> [w91]
        stop <- "stop" stop-if-true
        n93 = stacked-sequence {
          tunnel: w93 -> [w98 _]
          tunnel: [_ w99] -> _
          frame #0 {
            # "Delay loop?"
            n94 = To Double Precision Float(number=990) -> (double precision float=w96:dbl)
            n95 = Multiply(x=w98, y=w96) -> (x*y=w95:dbl)
            n96 = To Unsigned Long Integer(number=w95) -> (unsigned 32bit integer=w94:u32)
            n97 = Wait (ms)(milliseconds to wait=w94) -> ()  [unwired: 1 out]
          }
          frame #1 {
            n98 = local read "Running?"() -> (w100:bool)
            n99 = case shown="True" w100 {
              tunnel: [1 ("return type") w107] -> w99
              frame False {
              }
              frame True {
                w120 = 20 ("length")
                # "Collects Data From Card,\nSends It To The Chart"
                n100 = local read "bins"() -> (w125:u32)
                n101 = local read "Device ID"() -> (w133:u32)
                n102 = To Long Integer(number=w125) -> (32bit integer=w124:i32)
                n103 = local read "Number of Bins"() -> (w122:u32)
                n104 = dll-call lib="AmcsUsb.dll" fn="_AMCSUSB_DataStreamSize" label="DataStreamSize"("handle"=w133) -> ("return type"=w132:u16)  [unwired: 4 in, 2 out]
                n105 = expression code="x/2"(w132) -> (w131:u16)
                n106 = Subtract(x=w122, y=w120) -> (x-y=w121:u32)
                n107 = To Long Integer(number=w131) -> (32bit integer=w130:i32)
                n108 = Initialize Array(u32 0 ("element"), w130) -> (w134:u32[])
                n109 = dll-call lib="AmcsUsb.dll" fn="_AMCSUSB_ReadDataStream2" label="ReadDataStream2"("handle"=w133, "buffer"=w134, "BytesReturned"=u32 0) -> ("return type"=w107:i32, "buffer"=w126:u16[])  [unwired: 5 in, 2 out]
                "return type" <- w107
                n110 = stacked-sequence {
                  tunnel: w126 -> [w161 w178 w195 w212]
                  tunnel: w124 -> [w160 w166 w187 w204]
                  tunnel: [w149 _ _ _] -> w123
                  tunnel: [w148 _ _ _] -> w117
                  tunnel: w121 -> [w157 w174 w191 w208]
                  tunnel: w120 -> [w156 w175 w192 w209]
                  tunnel: [w154 _ _ _] -> w109
                  tunnel: "TC Start" -> [w153 w164 w181 w198]
                  tunnel: "TC Length" -> [w152 w165 w182 w199]
                  tunnel: [_ w172 _ _] -> w116
                  tunnel: [_ w169 _ _] -> w115
                  tunnel: [_ w168 _ _] -> w114
                  tunnel: [_ _ w185 _] -> w113
                  tunnel: [_ _ w184 _] -> w106
                  tunnel: [_ _ w183 _] -> w112
                  tunnel: [_ _ _ w202] -> w111
                  tunnel: [_ _ _ w201] -> w103
                  tunnel: [_ _ _ w200] -> w110
                  frame #0 {
                    n111 = Increment(x=0 ("dimension size")) -> (x+1=w146:i32)
                    n112 = Array Subset(array=w161, index=w146, length=w160) -> (w158:u16[])
                    n113 = To Double Precision Float(number=w158) -> (double precision float=w151:dbl[])
                    n114 = Array Subset(array=w151, index=w157, length=w156) -> (w159:dbl[])
                    n115 = call-poly <vilib>:"Mean.vi"("X"=w159) -> ("mean"=w150:dbl)  [unwired: 1 out]
                    n116 = Array Subset(array=w151, index=w153, length=w152) -> (w155:dbl[])
                    n117 = Add Array Elements(numeric array=w155) -> (sum=w154:dbl)
                    n118 = To Double Precision Float(number=w151) -> (double precision float=w149:dbl[])
                    n119 = Subtract(x=w149, y=w150) -> (x-y=w148:dbl[])
                  }
                  frame #1 {
                    n120 = Multiply(x=w166, y=1 ("Far Input Ch")) -> (x*y=w163:i32)
                    n121 = Increment(x=w163) -> (x+1=w162:i32)
                    n122 = Array Subset(array=w178, index=w162, length=w166) -> (w177:u16[])
                    n123 = To Double Precision Float(number=w177) -> (double precision float=w168:dbl[])
                    n124 = Array Subset(array=w168, index=w174, length=w175) -> (w176:dbl[])
                    n125 = call-poly <vilib>:"Mean.vi"("X"=w176) -> ("mean"=w170:dbl)  [unwired: 1 out]
                    n126 = To Double Precision Float(number=w168) -> (double precision float=w171:dbl[])
                    n127 = Array Subset(array=w168, index=w164, length=w165) -> (w173:dbl[])
                    n128 = Subtract(x=w171, y=w170) -> (x-y=w169:dbl[])
                    n129 = Add Array Elements(numeric array=w173) -> (sum=w172:dbl)
                  }
                  frame #2 {
                    n130 = Multiply(x=w187, y=2 ("Far Input Ch")) -> (x*y=w180:i32)
                    n131 = Increment(x=w180) -> (x+1=w179:i32)
                    n132 = Array Subset(array=w195, index=w179, length=w187) -> (w194:u16[])
                    n133 = To Double Precision Float(number=w194) -> (double precision float=w183:dbl[])
                    n134 = Array Subset(array=w183, index=w191, length=w192) -> (w193:dbl[])
                    n135 = call-poly <vilib>:"Mean.vi"("X"=w193) -> ("mean"=w188:dbl)  [unwired: 1 out]
                    n136 = To Double Precision Float(number=w183) -> (double precision float=w189:dbl[])
                    n137 = Array Subset(array=w183, index=w181, length=w182) -> (w190:dbl[])
                    n138 = Subtract(x=w189, y=w188) -> (x-y=w184:dbl[])
                    n139 = Add Array Elements(numeric array=w190) -> (sum=w185:dbl)
                  }
                  frame #3 {
                    n140 = Multiply(x=w204, y=3 ("Far Input Ch")) -> (x*y=w197:i32)
                    n141 = Increment(x=w197) -> (x+1=w196:i32)
                    n142 = Array Subset(array=w212, index=w196, length=w204) -> (w211:u16[])
                    n143 = To Double Precision Float(number=w211) -> (double precision float=w200:dbl[])
                    n144 = Array Subset(array=w200, index=w208, length=w209) -> (w210:dbl[])
                    n145 = call-poly <vilib>:"Mean.vi"("X"=w210) -> ("mean"=w205:dbl)  [unwired: 1 out]
                    n146 = To Double Precision Float(number=w200) -> (double precision float=w206:dbl[])
                    n147 = Array Subset(array=w200, index=w198, length=w199) -> (w207:dbl[])
                    n148 = Subtract(x=w206, y=w205) -> (x-y=w201:dbl[])
                    n149 = Add Array Elements(numeric array=w207) -> (sum=w202:dbl)
                  }
                }
                n150 = Equal To 0?(x=w107) -> (x = 0?=w108:bool)
                n151 = Multiply(x=w106, y="y") -> (x*y=w105:dbl[])
                n152 = Multiply(x=w103, y="y") -> (x*y=w102:dbl[])
                n153 = Build Array(w117, w115, w105, w102) -> (w129:dbl[][])
                n154 = Bundle(w109, w116, w113, w111) -> (w127:cluster{dbl, dbl, dbl, dbl})  [unwired: 1 in]
                n155 = Build Array(w123, w114, w112, w110) -> (w128:dbl[][])
                n156 = case shown="True" w108 {
                  tunnel: w129 -> [_ w145]
                  tunnel: w128 -> [_ w144]
                  tunnel: w127 -> [_ w143]
                  tunnel: w123 -> [_ w140]
                  tunnel: w114 -> [_ w137]
                  tunnel: w112 -> [_ w138]
                  tunnel: w110 -> [_ w139]
                  frame False {
                  }
                  frame True {
                    n157 = local read "Data Reads"() -> (w141:i32)
                    n158 = global write "Scalar_Data.vi" "Scalar Data"(w140) -> ()
                    n159 = global write "Scalar_Data_2.vi" "Scalar Data 2"(w137) -> ()
                    n160 = global write "Scalar_Data_3.vi" "Scalar Data 3"(w138) -> ()
                    n161 = global write "Scalar_Data_4.vi" "Scalar Data 4"(w139) -> ()
                    n162 = Increment(x=w141) -> (x+1=w142:i32)
                    n163 = local write "Data Reads"(w142) -> ()
                    "Corrected Return" <- w145
                    "Raw Uncorrected Return" <- w144
                    "Total Counts" <- w143
                  }
                }
              }
            }
          }
        }
        "Loop Count" <- w91
      }
    }
    frame #5 {
      # "Closes Any Open Cards\nAnd Resets Indicators\nOn Front Panel"
      n164 = dll-call lib="AmcsUsb.dll" fn="_AMCSUSB_Close_All" label="Close_All"() -> ()  [unwired: 4 in, 2 out]
      n165 = local write "Device ID"(u32 0 ("Device ID")) -> ()
      n166 = local write "Open?"(TRUE ("Open?")) -> ()
      n167 = local write "Running?"(FALSE ("Running?")) -> ()
    }
  }
